vi "Split Key.vi"(0 "Key":string) -> (2 "Type":string, 3 "ID":string)   [LabVIEW 2020, in "Volatus.lvlib" / "Identity.lvclass"]
uses:
  Identity.lvclass
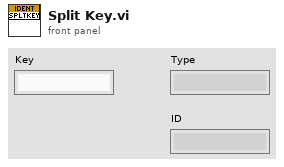
[diagram p1: front panel]
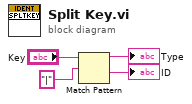
[diagram p0: block diagram]
diagram:
  n1 = Match Pattern(string="Key", regular expression="|") -> (before substring=→"Type":string, after substring=→"ID":string)  [unwired: 1 in, 2 out]
